vi "Change all tentative sn assignments to available.vi"(8 "Error in (no error)":errorcluster) -> (0 "Error out":errorcluster)   [LabVIEW 2013]
uses:
  Main Support/Global 2.vi
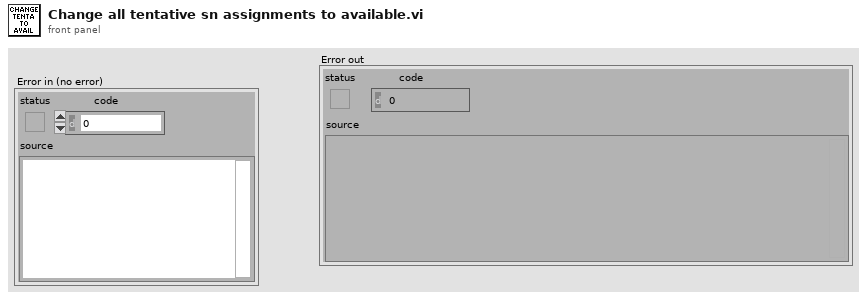
[diagram p1: front panel]
types:
  T1 = enum16{"get next serial number available", "change status to assigned", "change status to available", "change status to tentative"}
  T2 = enum16{"Query", "Insert", "Select", "Dump Recs", "Get Rec Count", "Get Col Names", "Insert all fields", "Find", "Get last test result", "Get work order qty", "Set work order qty", "Save test report", "Get test report", "Execute query no data", "Select count", "Query and return row 0 col 0"}
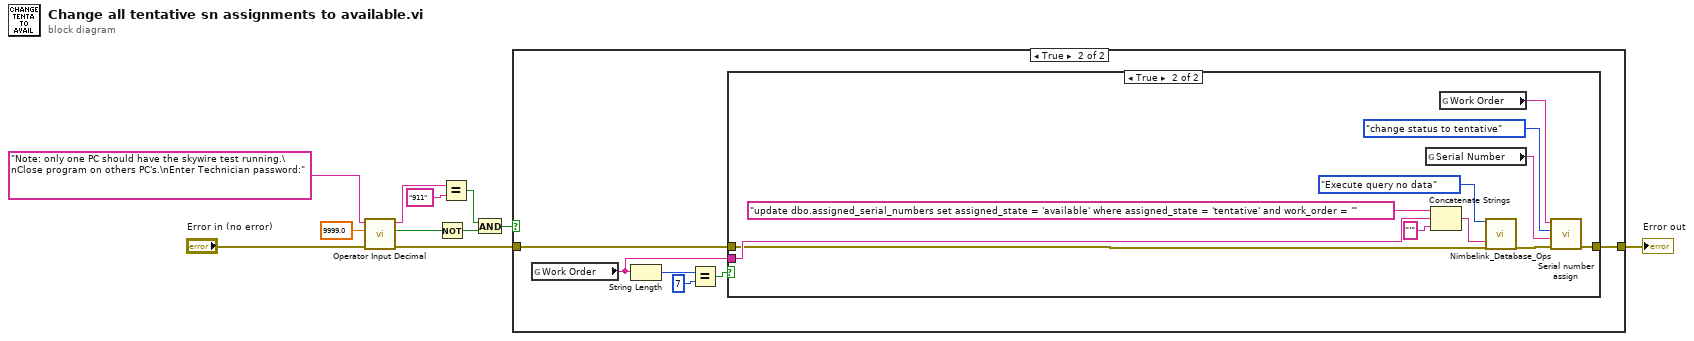
[diagram p0: block diagram]
diagram:
  n1 = call "Operator Input Decimal.vi"("error in (no error)"="Error in (no error)", "Upper limit"=9999.0, "Message"="Note: only one PC should have the skywire test running.\nClose program on others PC's.\nEnter Technician password:") -> ("error out"=w9:errorcluster, "Stop button hit"=w3:bool, "Response"=w8:string)  [unwired: 6 in]
  n2 = Not(x=w3) -> (.not. x?=w4:bool)
  n3 = Equal?(x=w8, y="911") -> (x = y?=w5:bool)
  n4 = And(x=w5, y=w4) -> (x .and. y?=w6:bool)
  n5 = case shown="True" w6 {
    tunnel: [w12 w18] -> w11
    tunnel: w9 -> [w12 w13]
    frame False {
    }
    frame True {
      n6 = global read "Global 2.vi" "Work Order"() -> (w17:string)
      n7 = String Length(string=w17) -> (length=w16:i32)
      n8 = Equal?(x=w16, y=7) -> (x = y?=w14:bool)
      n9 = case shown="True" w14 {
        tunnel: w17 -> [_ w28]
        tunnel: [w19 w23] -> w18
        tunnel: w13 -> [w19 w22]
        frame False {
        }
        frame True {
          n10 = global read "Global 2.vi" "Serial Number"() -> (w21:string)
          n11 = Concatenate Strings("update dbo.assigned_serial_numbers set assigned_state = 'available' where assigned_state = 'tentative' and work_order = '" ("string"), w28, "'" ("string")) -> (w26:string)
          n12 = global read "Global 2.vi" "Work Order"() -> (w20:string)
          n13 = call "Nimbelink_Database_Ops.vi"("Operation"=T2."Execute query no data", "SQL Query"=w26, "Error in (no error)"=w22) -> ("Error out"=w25:errorcluster)  [unwired: 9 in, 7 out]
          n14 = call "Serial number assign.vi"("Error in (no error)"=w25, "Serial number in"=w21, "Operation"=T1."change status to tentative", "Work order"=w20) -> ("Error out"=w23:errorcluster)  [unwired: 5 in, 2 out]
        }
      }
    }
  }
  "Error out" <- w11
